vi "Configure Square Wave Sweep Test.vi"(5 "Cycle Count (10)":i32=10, 6 "High-level Time (1 s)":dbl=1.0, 7 "Low-level Time (1 s)":dbl=1.0, 8 "error in (no error)":errorcluster, 9 "High-level Voltage (1)":dbl=1.0, 10 "Low-level Voltage (-1)":dbl=-1.0, 11 "VISA resource name":refnum<visa-resource-name>) -> (0 "error out":errorcluster, 3 "VISA resource name out":refnum<visa-resource-name>)   [LabVIEW 2020, in "Keithley 6517.lvlib"]
doc: "Sets the high-level voltage, high-level time, low-level voltage, low-level time and the cycle count for the square wave sweep test.\n\nNote:\nCall <b> Configure Test Sequence Common Characteristics </b> first to arm and configures the test sequence.\n\nThis VI is <B>NOT</B> compatible with model <B>6514</B>."
uses:
  <instrlib>/Keithley 6517/Keithley 6517.lvlib
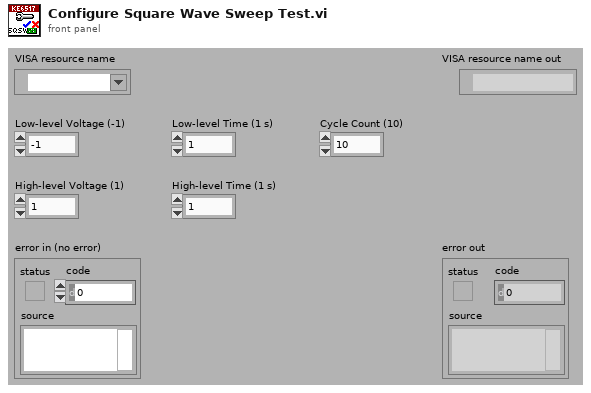
[diagram p1: front panel]
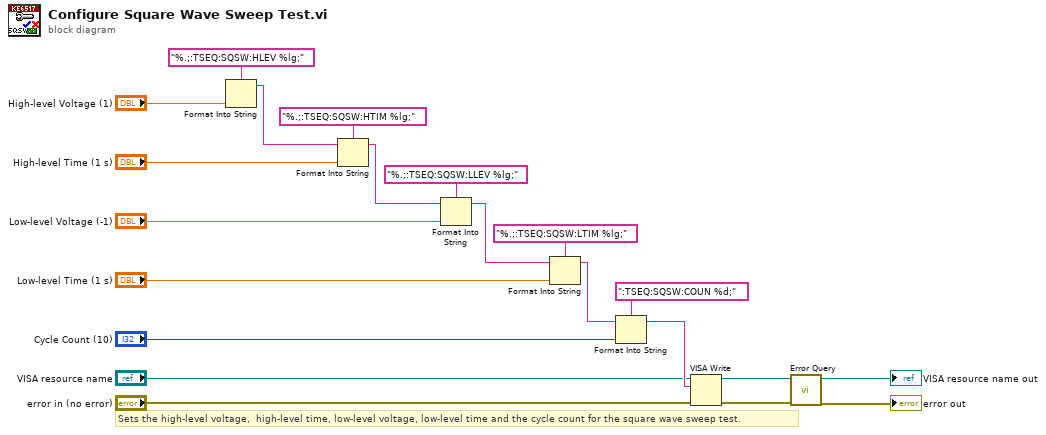
[diagram p0: block diagram]
diagram:
  # "Sets the high-level voltage,  high-level time, low-level voltage, low-level time and the cycle count for the square wave sweep test."
  n1 = Format Into String(format string="%.;:TSEQ:SQSW:HLEV %lg;", "High-level Voltage (1)") -> (resulting string=w19:string)  [unwired: 2 in, 1 out]
  n2 = Format Into String(format string="%.;:TSEQ:SQSW:HTIM %lg;", initial string=w19, "High-level Time (1 s)") -> (resulting string=w16:string)  [unwired: 1 in, 1 out]
  n3 = Format Into String(format string="%.;:TSEQ:SQSW:LLEV %lg;", initial string=w16, "Low-level Voltage (-1)") -> (resulting string=w13:string)  [unwired: 1 in, 1 out]
  n4 = Format Into String(format string="%.;:TSEQ:SQSW:LTIM %lg;", initial string=w13, "Low-level Time (1 s)") -> (resulting string=w10:string)  [unwired: 1 in, 1 out]
  n5 = Format Into String(format string=":TSEQ:SQSW:COUN %d;", initial string=w10, "Cycle Count (10)") -> (resulting string=w7:string)  [unwired: 1 in, 1 out]
  n6 = VISA Write(VISA resource name="VISA resource name", write buffer=w7, error in (no error)="error in (no error)") -> (VISA resource name out=w4:refnum<visa-resource-name>, error out=w3:errorcluster)  [unwired: 1 out]
  n7 = call <instrlib>:"Error Query.vi"("error in (no error)"=w3, "VISA resource name"=w4) -> ("error out"=→"error out":errorcluster, "VISA resource name out"=→"VISA resource name out":refnum<visa-resource-name>)  [unwired: 6 in, 2 out]
